vi "Gamma PID.vi"(6 "nonzero temperature":dbl=300.0, 10 "sweep folder path":path, 11 "adaptive parameters":T1={"peaks are known -- parameters"={"Def Gamma (kHz)"=0.5, "dV"=17.0, "time in Gamma (sec)"=7.0, "phi-star"=0.0, "all peaks (kHz)"=[], "delta t (sec)"=22.0, "default step (Hz)"=0.0, "all gamma (kHz)"=[564.0, 649.0, 987.0, 1133.0, 1214.0, 1585.0, 1763.0, 1823.0, 1880.0, 1899.0, 2032.0, 2138.0, 2221.0, 2270.0, 2350.0, 2456.0, 2580.0, 2634.0, 2831.0, 2960.0, 2965.0, 3131.0, 3328.0, 3469.0, 3553.0, 0.0, 3615.0, 3734.0, 0.0, 0.0, 0.0, 4236.0, 4300.0, 4331.0], "peaks OK"=FALSE, "gamma OK"=FALSE, "near omega (kHz)"=0.0, "near gamma (kHz)"=0.0, "min step (Hz)"=10000.0, "max step(Hz)"=0.01, "min gamma (kHz)"=0.01, "all time in gamma (sec)"=[]}, "find peak - parameters"={"wavepacket"={"R"=0.5, "wave number"=17.0, "delta k"=7.0, "radii vector"=[], "radial section"=[], "wave vector"=22.0, "wavepacket is"=TRUE}, "number of grid points"=70, "decimation threshold"=1, "Voltage range"=0.1, "target freq step"=20.0, "target spot size"=0.05, "factor"=1.0, "another factor"=1.0, "analyze last # sec"=3, "scale factor"=3}} {"find peak - parameters"."wavepacket"."delta k" format="%#_3f"; "find peak - parameters"."wavepacket"."wave number" format="%#_3f"; "find peak - parameters"."wavepacket"."R" format="%#_3f"}) -> (3 "adaptive parameters out":T1={"peaks are known -- parameters"={"Def Gamma (kHz)"=0.5, "dV"=17.0, "time in Gamma (sec)"=7.0, "phi-star"=0.0, "all peaks (kHz)"=[], "delta t (sec)"=22.0, "default step (Hz)"=0.0, "all gamma (kHz)"=[564.0, 649.0, 987.0, 1133.0, 1214.0, 1585.0, 1763.0, 1823.0, 1880.0, 1899.0, 2032.0, 2138.0, 2221.0, 2270.0, 2350.0, 2456.0, 2580.0, 2634.0, 2831.0, 2960.0, 2965.0, 3131.0, 3328.0, 3469.0, 3553.0, 0.0, 3615.0, 3734.0, 0.0, 0.0, 0.0, 4236.0, 4300.0, 4331.0], "peaks OK"=FALSE, "gamma OK"=FALSE, "near omega (kHz)"=0.0, "near gamma (kHz)"=0.0, "min step (Hz)"=10000.0, "max step(Hz)"=0.01, "min gamma (kHz)"=0.01, "all time in gamma (sec)"=[]}, "find peak - parameters"={"wavepacket"={"R"=0.5, "wave number"=17.0, "delta k"=7.0, "radii vector"=[], "radial section"=[], "wave vector"=22.0, "wavepacket is"=TRUE}, "number of grid points"=70, "decimation threshold"=1, "Voltage range"=0.1, "target freq step"=20.0, "target spot size"=0.05, "factor"=1.0, "another factor"=1.0, "analyze last # sec"=3, "scale factor"=3}} {"find peak - parameters"."wavepacket"."delta k" format="%#_3f"; "find peak - parameters"."wavepacket"."wave number" format="%#_3f"; "find peak - parameters"."wavepacket"."R" format="%#_3f"})   [LabVIEW 2012]
uses:
  single sweep - adaptive parameters.ctl
  next chunk -- parameters.ctl
  find peak -- parameters.ctl
  wavepacket.ctl
  ctl -- name dispatcher -- action.ctl
  next chunk - read-write freq PID file - atomic actions .vi
  ctl -- name dispatcher.vi
  file -- 9w path.vi
  array -- find index - real.vi
  array -- interpolate -- i.vi
  Q -- check range -- i -- real.vi
  Q - not nan -- real.vi
  <vilib>/Utility/libraryn.llb/Check if File or Folder Exists.vi
  file -- read list of lines.vi
  parse -- find first line.vi
  parse -- get list of matches -- numbers.vi
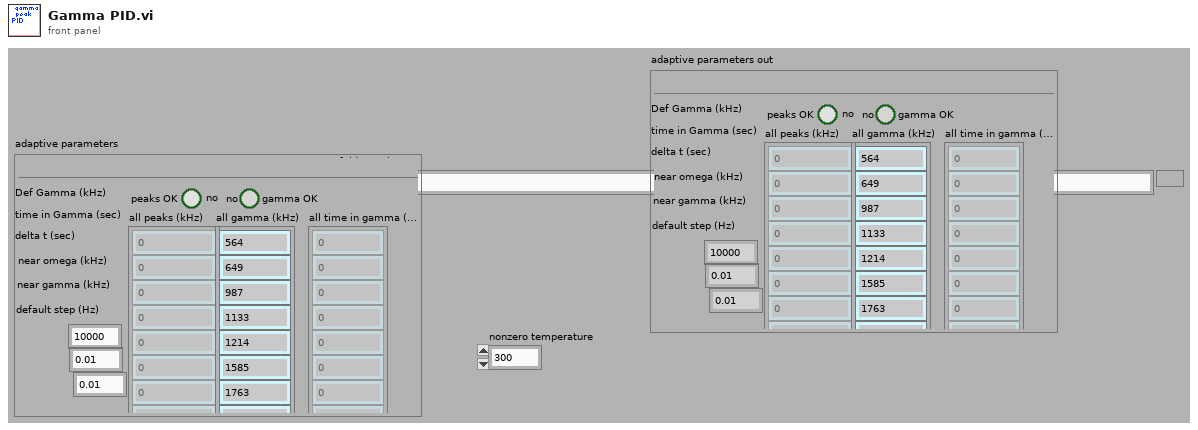
[diagram p1: front panel]
types:
  T1 = typedef "single sweep - adaptive parameters.ctl" = cluster{"peaks are known -- parameters":T2, "find peak - parameters":T3}
  T2 = typedef "next chunk -- parameters.ctl" = cluster{"Def Gamma (kHz)":dbl, "dV":dbl, "time in Gamma (sec)":dbl, "phi-star":dbl, "all peaks (kHz)":dbl[], "delta t (sec)":dbl, "default step (Hz)":dbl, "all gamma (kHz)":dbl[], "peaks OK":bool, "gamma OK":bool, "near omega (kHz)":dbl, "near gamma (kHz)":dbl, "min step (Hz)":dbl, "max step(Hz)":dbl, "min gamma (kHz)":dbl, "all time in gamma (sec)":dbl[]}
  T3 = typedef "find peak -- parameters.ctl" = cluster{"wavepacket":T4, "number of grid points":i32, "decimation threshold":i32, "Voltage range":dbl, "target freq step":dbl, "target spot size":dbl, "factor":dbl, "another factor":dbl, "analyze last # sec":i32, "scale factor":i32}
  T4 = typedef "wavepacket.ctl" = cluster{"R":dbl, "wave number":dbl, "delta k":dbl, "radii vector":dbl[], "radial section":cdb[], "wave vector":dbl, "wavepacket is":bool}
  T5 = typedef "ctl -- name dispatcher -- action.ctl" = enum16{"peak frequency", "peak frequency DUMP", "peak gamma DUMP", "peak gamma", "peak frequency TEST", "peak gamma TEST", "ultrasonic power", "time in gamma", "set temperature ", "set temperature timer", "peak default gamma", "last scan file", "peak freq gamma TEST", "peak NAMES", "errors", "P_I_D", "P", "I", "D", "power vs time", "power vs time TIMER", "void", "power log", "set temperature - SINE", "itc ltc log", "peak - time in gamma"}
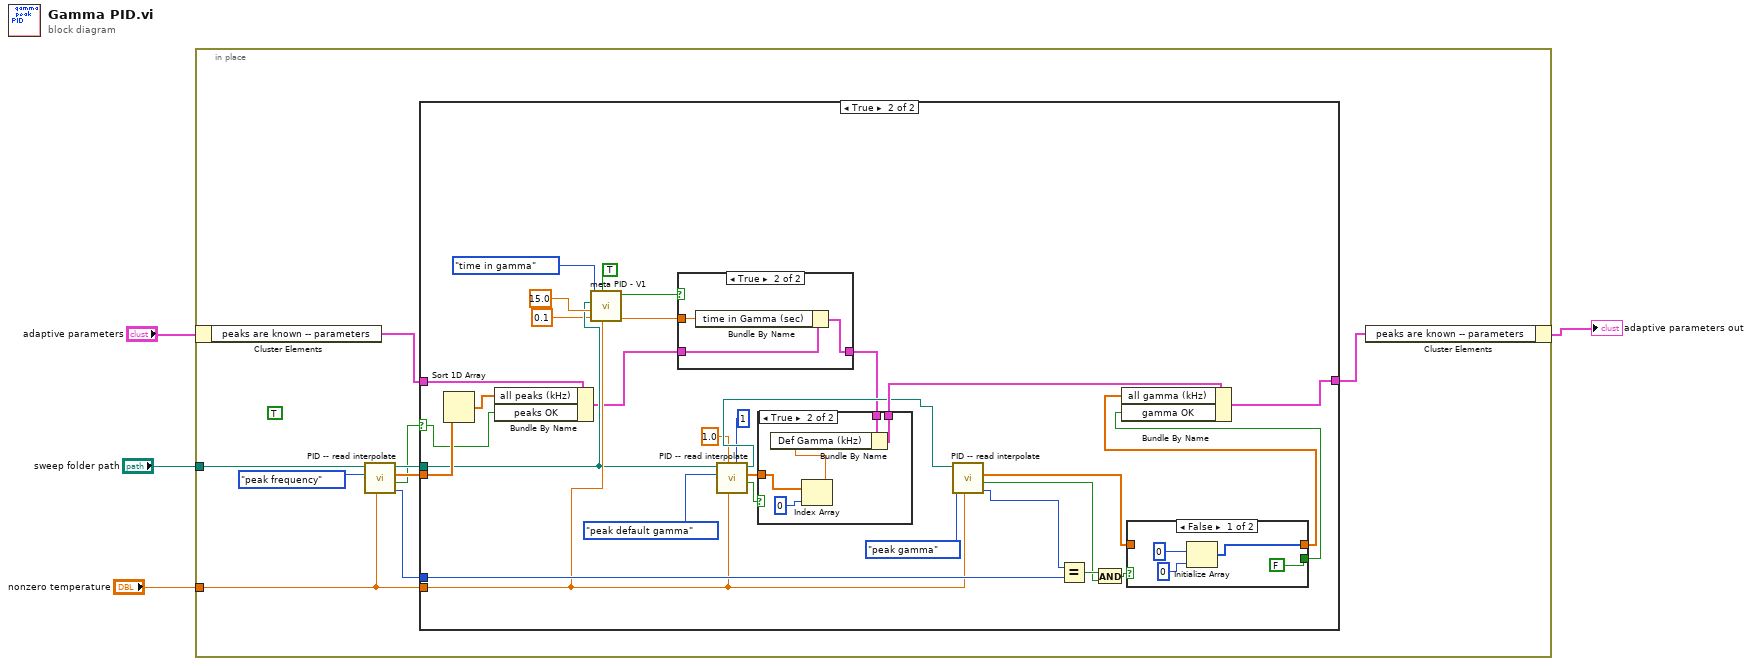
[diagram p0: block diagram]
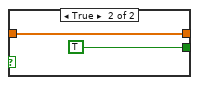
[diagram p5: hidden frame]
diagram:
  n1 = in-place {
    in-place-border: "sweep folder path" -> [w9]
    in-place-border: "nonzero temperature" -> [w8]
    (unwired) TRUE ("peaks are known -- parameters.peaks OK")
    n2 = in-place-cluster #1("adaptive parameters") -> ("peaks are known -- parameters"=w5:T2)
    n3 = call "PID -- read interpolate.vi"("temperature"=w8, "ctl PID file IN"=ctl_--_name_dispatcher_--_action."peak frequency", "sweep folder path"=w9) -> ("length out"=w11:i32, "PID OK !"=w7:bool, "PID freq"=w10:dbl[], "sweep folder path out"=w12:path)  [unwired: 4 in, 1 out]
    n4 = case shown="True" w7 {
      selector: w7 -> [_ w28]
      tunnel: w12 -> [_ w25]
      tunnel: w11 -> [_ w43]
      tunnel: w5 -> [w14 w42]
      tunnel: [w14 w41] -> w6
      tunnel: w10 -> [_ w30]
      tunnel: w8 -> [_ w26]
      frame False {
      }
      frame True {
        n5 = Sort 1D Array(array=w30) -> (sorted array=w29:dbl[])
        n6 = Bundle By Name(cluster=w42, "all peaks (kHz)"=w29, "peaks OK"=w28) -> (w21:T2)
        n7 = call "meta PID - V1.vi"("input parameter"=w26, "control?"=TRUE ("control power PID?"), "lower limit"=0.1 ("lower"), "upper limit"=15.0 ("upper"), "sweep folder path"=w25, "ctl name dispatch"=ctl_--_name_dispatcher_--_action."time in gamma") -> ("bezier output"=w22:dbl, "ok"=w23:bool)  [unwired: 2 in, 2 out]
        n8 = case shown="True" w23 {
          tunnel: w21 -> [w46 w48]
          tunnel: w22 -> [_ w49]
          tunnel: [w46 w47] -> w20
          frame False {
          }
          frame True {
            n9 = Bundle By Name(cluster=w48, "time in Gamma (sec)"=w49) -> (w47:T2)
          }
        }
        n10 = call "PID -- read interpolate.vi"("length"=1, "temperature"=w26, "default"=1.0, "ctl PID file IN"=ctl_--_name_dispatcher_--_action."peak default gamma", "sweep folder path"=w25) -> ("PID OK !"=w31:bool, "PID freq"=w40:dbl[], "sweep folder path out"=w44:path)  [unwired: 2 in, 2 out]
        n11 = case shown="True" w31 {
          tunnel: w20 -> [w50 w55]
          tunnel: [w50 w54] -> w45
          tunnel: w40 -> [_ w51]
          frame False {
          }
          frame True {
            n12 = Index Array(array=w51, index=0) -> (element=w52:dbl)
            n13 = Bundle By Name(cluster=w55, "Def Gamma (kHz)"=w52) -> (w54:T2)
          }
        }
        n14 = call "PID -- read interpolate.vi"("temperature"=w26, "ctl PID file IN"=ctl_--_name_dispatcher_--_action."peak gamma", "sweep folder path"=w44) -> ("length out"=w15:i32, "PID OK !"=w32:bool, "PID freq"=w35:dbl[])  [unwired: 4 in, 2 out]
        n15 = Equal?(x=w15, y=w43) -> (x = y?=w33:bool)
        n16 = And(x=w33, y=w32) -> (x .and. y?=w34:bool)
        n17 = case shown="False" w34 {
          tunnel: [w56 w61] -> w37
          tunnel: w35 -> [_ w61]
          tunnel: [FALSE ("peaks are known -- parameters.peaks OK") TRUE ("peaks are known -- parameters.peaks OK")] -> w36
          frame False {
            n18 = Initialize Array(0 ("index"), 0 ("index")) -> (w56:i32[])
          }
          frame True {
          }
        }
        n19 = Bundle By Name(cluster=w45, "all gamma (kHz)"=w37, "gamma OK"=w36) -> (w41:T2)
      }
    }
    n20 = in-place-cluster #1("peaks are known -- parameters"=w6) -> (→"adaptive parameters out":T1)
  }
